vi "Generate Saw_1wave.vi"(3 "start":dbl, 5 "finish":dbl) -> (1 "V out x":dbl[](array[numeric]))   [LabVIEW 2013]
uses:
  <vilib>/measure/NI_MABase.lvlib
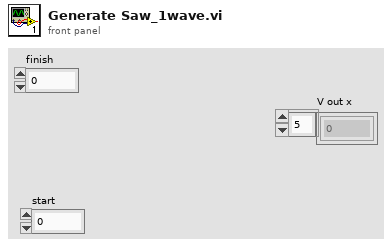
[diagram p1: front panel]
types:
  T1 = enum16{"Sine Wave", "Triangle Wave", "Square Wave", "Sawtooth Wave"}
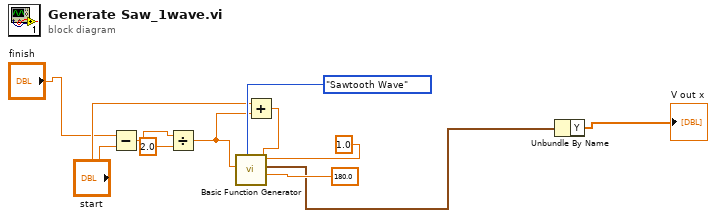
[diagram p0: block diagram]
diagram:
  n1 = Subtract(x="finish", y="start") -> (x-y=w7:dbl)
  n2 = Divide(x=w7, y=2.0) -> (x/y=w5:dbl)
  n3 = Add(x="start", y=w5) -> (x+y=w4:dbl)
  n4 = call <vilib>:"Basic Function Generator.vi"("offset"=w4, "signal type"=T1."Sawtooth Wave", "phase"=180.0, "amplitude"=w5, "frequency"=1.0) -> ("signal out"=w3:waveform(dbl))  [unwired: 4 in, 2 out]
  n5 = Unbundle By Name(w3) -> ("Y"=→"V out x":dbl[])
